vi "Auto Shooter Mode.vi"(0 "Unstuck Delay":dbl, 1 "Shooter Commands":T2, 2 "Shot Type":T3, 5 "Warmup Delay":dbl, 7 "RPM Tolerance":dbl, 9 "Faster Time":dbl, 11 "Initial RPM Increase":dbl, 12 "Current RPM":dbl, 13 "Shooter Presets":T1 {"Shooter PID Gains"."D" format="%.3f"; "Shooter PID Gains"."I" format="%.3f"; "Shooter PID Gains"."P" format="%.3f"}, 14 "Hopper Filled?":bool) -> (6 "Shoot State":T2, 8 "Hopper Speed":dbl, 10 "Wheel RPM":dbl)   [LabVIEW 2016]
uses:
  Common Code/Shooter Commands.ctl
  Common Code/Shot Type.ctl
  Common Code/Shooter Presets.ctl
  Common Code/Utilities/Change Detect Int.vi
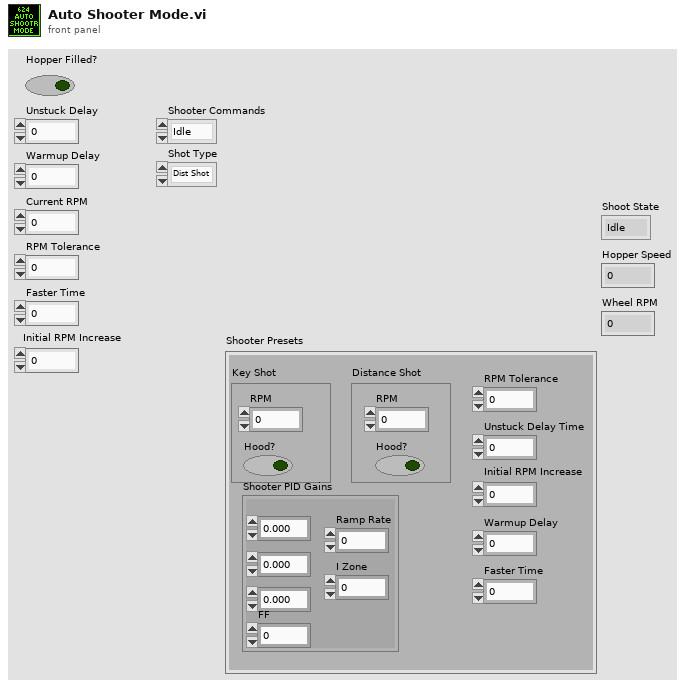
[diagram p1: front panel]
types:
  T1 = typedef "Shooter Presets.ctl" = cluster{"Key Shot":cluster{"RPM ":dbl, "Hood?":bool}, "Distance Shot":cluster{"RPM":dbl, "Hood?":bool}, "RPM Tolerance":dbl, "Unstuck Delay Time ":dbl, "Initial RPM Increase":dbl, "Warmup Delay":dbl, "Faster Time":dbl, "Shooter PID Gains":cluster{"P":dbl, "I":dbl, "D":dbl, "FF":dbl, "Ramp Rate":dbl, "I Zone":dbl}}
  T2 = typedef "Shooter Commands.ctl" = enum16{"Idle ", "Warmup ", "Shoot"}
  T3 = typedef "Shot Type.ctl" = enum16{"Dist Shot", "Key Shot"}
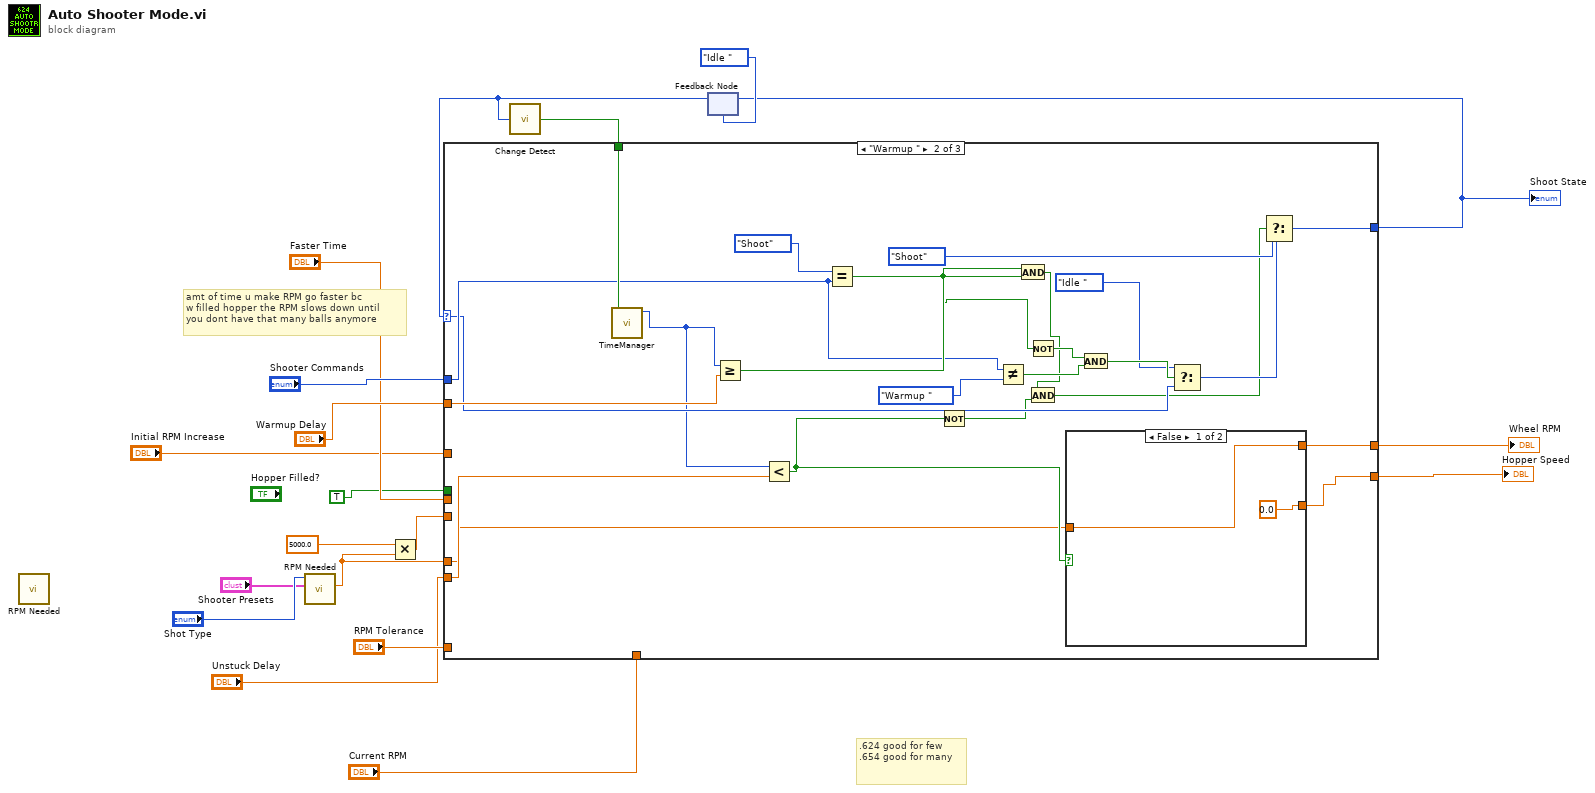
[diagram p0: block diagram]
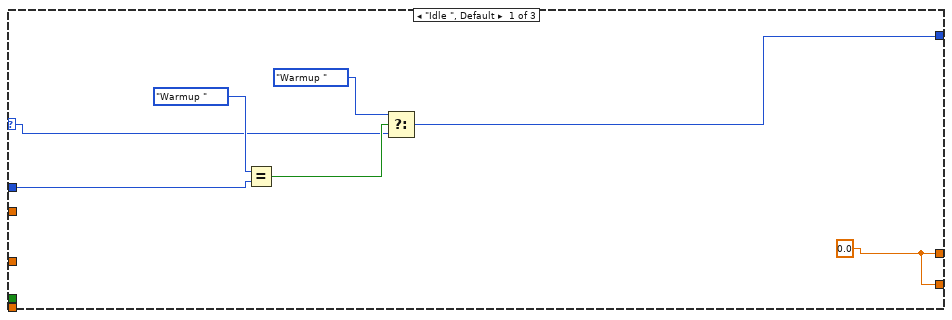
[diagram p2: hidden frame]
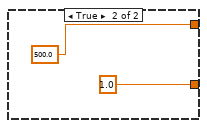
[diagram p3: hidden frame]
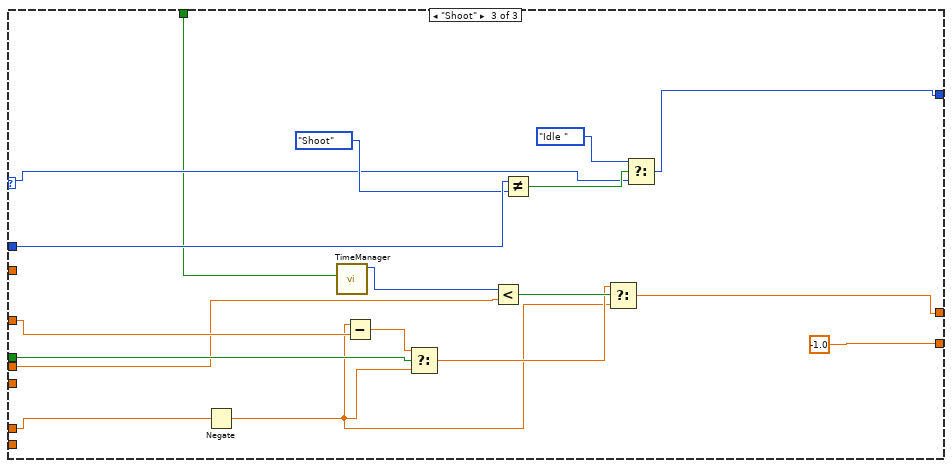
[diagram p4: hidden frame]
diagram:
  # "amt of time u make RPM go faster bc \nw filled hopper the RPM slows down until\nyou dont have that many balls anymore"
  # ".624 good for few\n.654 good for many"
  n1 = call "RPM Needed.vi"() -> ()  [unwired: 10 in, 2 out]
  n2 = call "RPM Needed.vi"("Shooter Presets"="Shooter Presets", "Shot Type"="Shot Type") -> ("RPM"=w6:dbl)  [unwired: 8 in, 1 out]
  n3 = Multiply(x=5000.0, y=w6) -> (x*y=w9:dbl)
  n4 = feedback #1(Shooter_Commands."Idle " ("Shooter Commands")) -> (w14:T2)
  n5 = call-poly "Change Detect.vi"("In"=w14) -> ("Changed?"=w13:bool)
  n6 = case shown="\"Warmup \"" w14 {
    selector: w14 -> [w20 w37 w68]
    tunnel: [w23 w48 w67] -> w17
    tunnel: "Shooter Commands" -> [w21 w44 w72]
    tunnel: "Unstuck Delay" -> [_ w35 _]
    tunnel: [w22 w29 w65] -> w8
    tunnel: [w22 w28 -1.0] -> w15
    tunnel: "Faster Time" -> [_ _ w57]
    tunnel: w13 -> [_ w47 w63]
    tunnel: "Current RPM" -> [_ _ _]
    tunnel: "Warmup Delay" -> [_ w45 _]
    tunnel: w9 -> [_ _ _]
    tunnel: w6 -> [_ w27 w56]
    tunnel: "RPM Tolerance" -> [_ _ _]
    tunnel: "Initial RPM Increase" -> [_ _ w64]
    tunnel: TRUE -> [_ _ w59]
    frame "Idle ", Default {
      w22 = 0.0
      n7 = Equal?(x=Shooter_Commands."Warmup " ("Shooter Commands"), y=w21) -> (x = y?=w25:bool)
      n8 = Select(t=Shooter_Commands."Warmup " ("Shooter Commands"), s=w25, f=w20) -> (s? t:f=w23:T2)
    }
    frame "Warmup " {
      n9 = call "TimeManager.vi"("Reset?"=w47) -> ("Time Since Reset"=w31:u32)  [unwired: 9 in, 1 out]
      n10 = Greater Or Equal?(x=w31, y=w45) -> (x >= y?=w46:bool)
      n11 = Less?(x=w31, y=w35) -> (x < y?=w30:bool)
      n12 = Equal?(x=Shooter_Commands."Shoot" ("Shooter Commands"), y=w44) -> (x = y?=w40:bool)
      n13 = Not(x=w30) -> (.not. x?=w34:bool)
      n14 = Not Equal?(x=w44, y=Shooter_Commands."Warmup " ("Shooter Commands")) -> (x != y?=w42:bool)
      n15 = And(x=w40, y=w46) -> (x .and. y?=w32:bool)
      n16 = Not(x=w40) -> (.not. x?=w41:bool)
      n17 = And(x=w32, y=w34) -> (x .and. y?=w33:bool)
      n18 = case shown="False" w30 {
        tunnel: [w52 500.0] -> w29
        tunnel: [0.0 1.0] -> w28
        tunnel: w27 -> [w52 _]
        frame False {
        }
        frame True {
        }
      }
      n19 = And(x=w41, y=w42) -> (x .and. y?=w39:bool)
      n20 = Select(t=Shooter_Commands."Idle " ("Shooter Commands"), s=w39, f=w37) -> (s? t:f=w36:T2)
      n21 = Select(t=Shooter_Commands."Shoot" ("Shooter Commands"), s=w33, f=w36) -> (s? t:f=w48:T2)
    }
    frame "Shoot" {
      n22 = Negate(x=w56) -> (-x=w55:dbl)
      n23 = call "TimeManager.vi"("Reset?"=w63) -> ("Time Since Reset"=w62:u32)  [unwired: 9 in, 1 out]
      n24 = Subtract(x=w55, y=w64) -> (x-y=w58:dbl)
      n25 = Select(t=w58, s=w59, f=w55) -> (s? t:f=w60:dbl)
      n26 = Less?(x=w62, y=w57) -> (x < y?=w61:bool)
      n27 = Not Equal?(x=w72, y=Shooter_Commands."Shoot" ("Shooter Commands")) -> (x != y?=w70:bool)
      n28 = Select(t=w60, s=w61, f=w55) -> (s? t:f=w65:dbl)
      n29 = Select(t=Shooter_Commands."Idle " ("Shooter Commands"), s=w70, f=w68) -> (s? t:f=w67:T2)
    }
  }
  "Wheel RPM" <- w8
  "Hopper Speed" <- w15
  "Shoot State" <- w17
  n30 = feedback-in #1(w17) -> ()
